vi "DiscoverDevices.vi"(6 "wait for reply (T)":bool=TRUE, 8 "error in":errorcluster) -> (0 "error out":errorcluster, 1 "timed out?":bool, 2 "CCDs":refnum<class "CCD.lvclass">[](array[class]), 3 "Monos":refnum<class "Monochromator.lvclass">[](array[class]), 5 "SCDs":refnum<class "SCD.lvclass">[](array[class]))   [LabVIEW 2023, in "DeviceManager.lvlib"]
doc: "Requests from the ICL to discover monochromators, cameras and single channel detectors.\n_____\nCreated using DQMH Event Scripter 7.0.0.1280."
uses:
  DeviceManager.lvlib
  Classes/Mono/Monochromator.lvclass
  Classes/CCD/CCD.lvclass
  Classes/SCD/SCD.lvclass
  DiscoverDevices Argument--cluster.ctl
  DiscoverDevices (Reply Payload)--cluster.ctl
panel:
  # "Connector Pane"
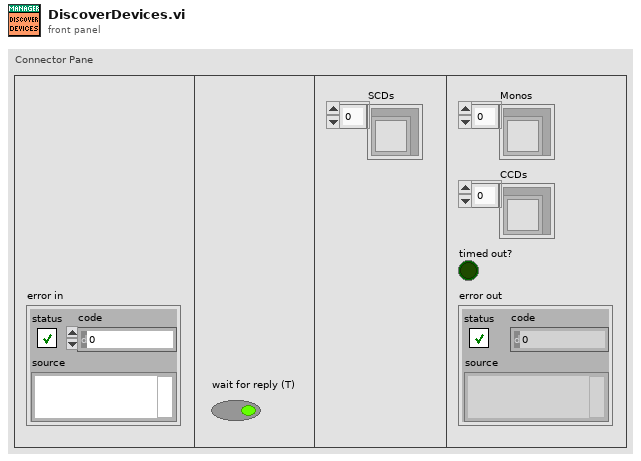
[diagram p1: front panel]
types:
  T1 = typedef "DeviceManager.lvlib/DiscoverDevices Argument--cluster.ctl" = cluster{"Wait Notifier":refnum<notifier>, "wait for reply":bool}
  T2 = typedef "DeviceManager.lvlib/Request Events--cluster.ctl" = cluster{"Stop Module":refnum<user-event>, "Show Panel":refnum<user-event>, "Hide Panel":refnum<user-event>, "Get Module Execution Status":refnum<user-event>, "Show Diagram":refnum<user-event>, "StartICL":refnum<user-event>, "OpenWebSocketCommunication":refnum<user-event>, "Private":cluster{"ICLstartNotification":refnum<user-event>}, "ICLshutdown":refnum<user-event>, "SendJSONandAskForReply":refnum<user-event>, "DiscoverDevices":refnum<user-event>}
  T3 = typedef "DeviceManager.lvlib/DiscoverDevices (Reply Payload)--cluster.ctl" = cluster{"Monos":refnum<class "Monochromator.lvclass">[], "CCDs":refnum<class "CCD.lvclass">[], "SCDs":refnum<class "SCD.lvclass">[], "error":errorcluster}
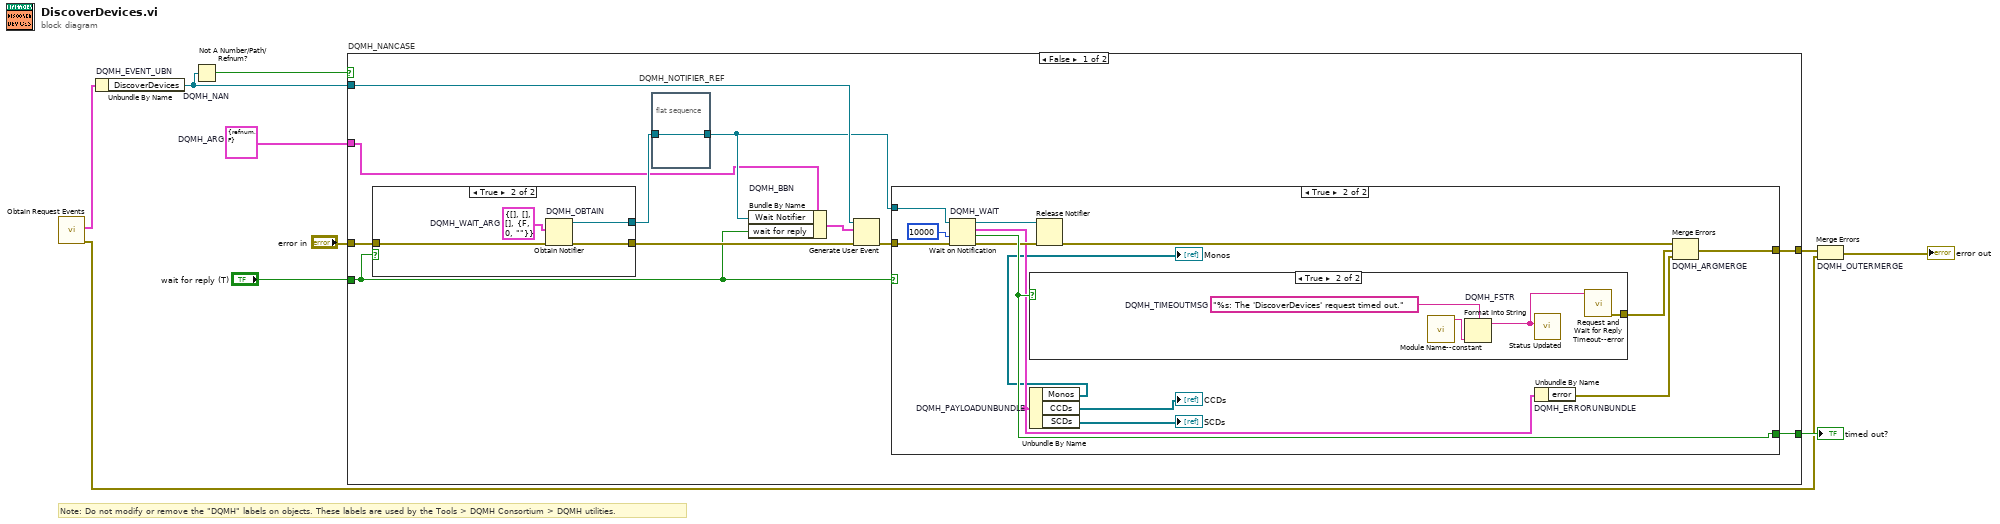
[diagram p0: block diagram]
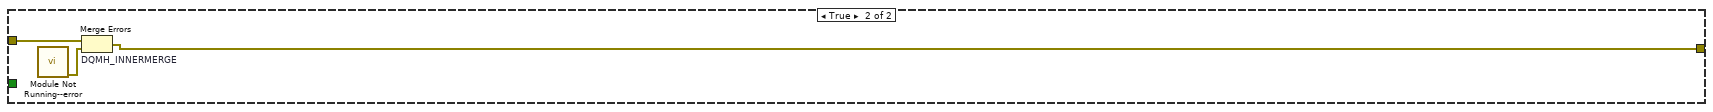
[diagram p5: hidden frame]
diagram:
  w4 = T1 {"Wait Notifier"=refnum, "wait for reply"=FALSE}  # DQMH_ARG
  # "Note: Do not modify or remove the \"DQMH\" labels on objects. These labels are used by the Tools > DQMH Consortium > DQMH utilities."
  n1 = call "Obtain Request Events.vi"() -> ("error out"=w2:errorcluster, "DeviceManager Request Events"=w1:T2)  [unwired: 10 in]
  n2 = Unbundle By Name "DQMH_EVENT_UBN"(w1) -> ("DiscoverDevices"=w8:refnum<user-event>)
  n3 = Not A Number/Path/Refnum? "DQMH_NAN"(number/path/refnum=w8) -> (NaN/Path/Refnum?=w7:bool)
  n4 = case "DQMH_NANCASE" shown="False" w7 {
    tunnel: "error in" -> [w21 w49]
    tunnel: w8 -> [w19 _]
    tunnel: [w16 w48] -> w5
    tunnel: [w17 _] -> w6
    tunnel: w4 -> [w12 _]
    tunnel: "wait for reply (T)" -> [w11 _]
    frame False {
      n5 = case shown="True" w11 {
        tunnel: w21 -> [w42 w46]
        tunnel: [w42 w45] -> w18
        tunnel: [_ w43] -> w14
        frame False {
        }
        frame True {
          w44 = T3 {"Monos"=[], "CCDs"=[], "SCDs"=[], "error"={"status"=FALSE, "code"=0, "source"=""}}  # DQMH_WAIT_ARG
          n6 = Obtain Notifier "DQMH_OBTAIN"(notification data type=w44, error in (no error)=w46) -> (notifier out=w43:refnum<notifier>, error out=w45:errorcluster)  [unwired: 2 in, 1 out]
        }
      }
      n7 = flat-sequence "DQMH_NOTIFIER_REF" {
        tunnel: w14 -> [w22]
        tunnel: [w22] -> w13
        frame #0 {
        }
      }
      n8 = Bundle By Name "DQMH_BBN"(cluster=w12, "Wait Notifier"=w13, "wait for reply"=w11) -> (w15:T1)
      n9 = Generate User Event(user event=w19, event data cluster=w15, error in=w18) -> (error out=w20:errorcluster)  [unwired: 1 in, 1 out]
      n10 = case shown="True" w11 {
        tunnel: w20 -> [w23 w37]
        tunnel: w13 -> [_ w36]
        tunnel: [_ w34] -> w17
        tunnel: [w23 w33] -> w16
        frame False {
        }
        frame True {
          n11 = Wait on Notification "DQMH_WAIT"(notifier=w36, timeout in ms (-1)=10000, error in (no error)=w37) -> (notifier out=w35:refnum<notifier>, notification=w28:T3, timed out?=w34:bool, error out=w32:errorcluster)  [unwired: 1 in]
          n12 = case shown="True" w34 {
            tunnel: [_ w39] -> w29
            frame False {
            }
            frame True {
              w41 = "%s: The 'DiscoverDevices' request timed out."  # DQMH_TIMEOUTMSG
              n13 = call "Module Name--constant.vi"() -> ("Module Name"=w38:string)  [unwired: 11 in]
              n14 = Format Into String "DQMH_FSTR"(format string=w41, w38) -> (resulting string=w40:string)  [unwired: 2 in, 1 out]
              n15 = call "Status Updated.vi"("Status"=w40) -> ()  [unwired: 10 in, 1 out]
              n16 = call "Request and Wait for Reply Timeout--error.vi"("Error Message"=w40) -> ("error out"=w39:errorcluster)  [unwired: 10 in]
            }
          }
          n17 = Unbundle By Name "DQMH_PAYLOADUNBUNDLE"(w28) -> ("Monos"=→"Monos":refnum<class "Monochromator.lvclass">[], "CCDs"=→"CCDs":refnum<class "CCD.lvclass">[], "SCDs"=→"SCDs":refnum<class "SCD.lvclass">[])
          n18 = Release Notifier(notifier=w35, error in (no error)=w32) -> (error out=w31:errorcluster)  [unwired: 1 in, 2 out]
          n19 = Unbundle By Name "DQMH_ERRORUNBUNDLE"(w28) -> ("error"=w30:errorcluster)
          n20 = Merge Errors "DQMH_ARGMERGE"(w31, w29, w30) -> (w33:errorcluster)
        }
      }
    }
    frame True {
      n21 = call "Module Not Running--error.vi"() -> ("error out"=w47:errorcluster)  [unwired: 11 in]
      n22 = Merge Errors "DQMH_INNERMERGE"(w49, w47) -> (w48:errorcluster)
    }
  }
  "timed out?" <- w6
  n23 = Merge Errors "DQMH_OUTERMERGE"(w5, w2) -> (→"error out":errorcluster)
